vi "API - Get Rx Channels.vi"(7 "MCLB":refnum<vi>, 8 "error in (no error)":errorcluster, 11 "Node Ptr":T1 format="%.0x") -> (0 "error out":errorcluster, 3 "Node Ptr out":T1 format="%.0x", 5 "Channel Info":string[][](array[string]))   [LabVIEW 2016, in "UDP-Custom-Device System Explorer.lvlib"]
uses:
  UDP-Custom-Device System Explorer.lvlib
  <vilib>/NI Veristand/Custom Device API/Custom Device Item Ref.ctl
  Types/Channel Data Type.ctl
  Shared/Constants.vi
  <vilib>/NI Veristand/Custom Device API/Get Item Property (U16).vi
  <vilib>/NI VeriStand/Custom Device API/Custom Device API.lvlib
  Shared/UDP-Custom-Device Shared.lvlib
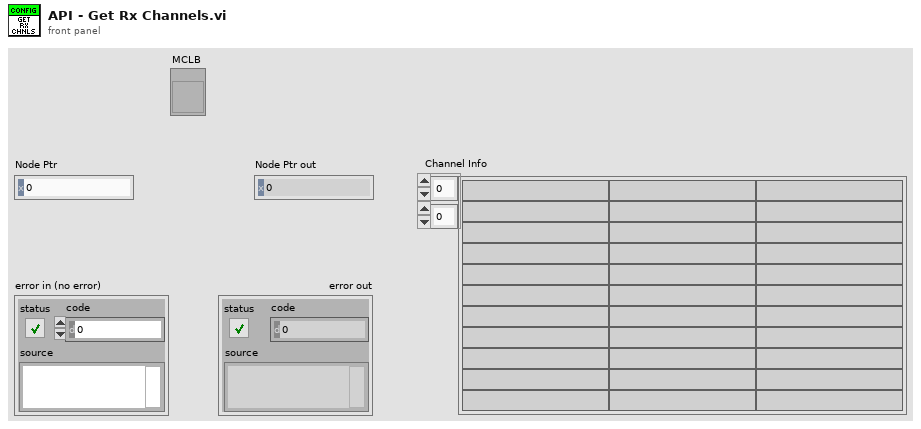
[diagram p1: front panel]
types:
  T1 = typedef "Custom Device API.lvlib/Custom Device Item Ref.ctl" = u64
  T2 = typedef "Custom Device API.lvlib/Custom Device Item Info.ctl" = cluster{"Name":string, "Is Channel":bool, "GUID":string, "Is Waveform":bool}
  T3 = typedef "UDP-Custom-Device System Explorer.lvlib/Channel Data Type.ctl" = enum16{"Boolean", "Single"}
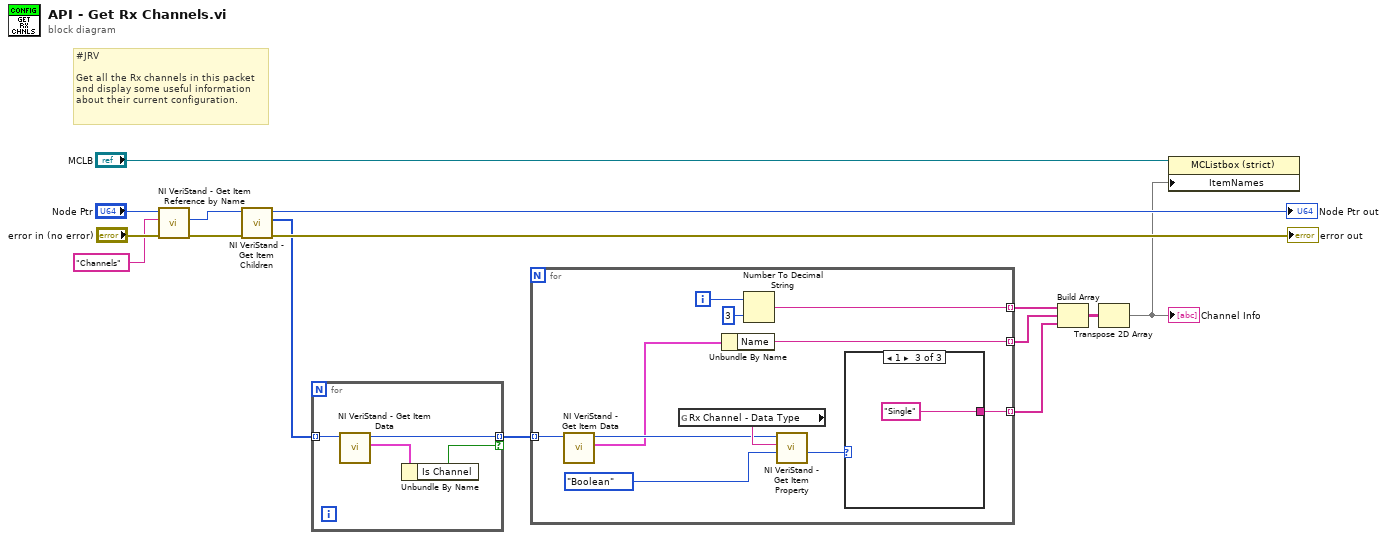
[diagram p0: block diagram]
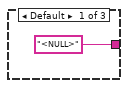
[diagram p2: hidden frame]
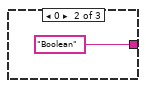
[diagram p3: hidden frame]
diagram:
  # "#JRV\n\nGet all the Rx channels in this packet\nand display some useful information\nabout their current configuration."
  n1 = call <vilib>:"NI VeriStand - Get Item Reference by Name.vi"("error in (no error)"="error in (no error)", "Item Name"="Channels" ("Section Name"), "Parent Ref in"="Node Ptr") -> ("error out"=w2:errorcluster, "Item Ref"=w4:T1)  [unwired: 5 in, 2 out]
  n2 = call <vilib>:"NI VeriStand - Get Item Children.vi"("error in (no error)"=w2, "Item Ref in"=w4) -> ("error out"=→"error out":errorcluster, "Child Refs"=w6:T1[], "Item Ref out"=→"Node Ptr out":T1)  [unwired: 6 in, 1 out]
  n3 = for {
    tunnel: [w18] -> w7 mode=indexing if=w16
    tunnel: w6 -> [w19] mode=indexing
    n4 = call <vilib>:"NI VeriStand - Get Item Data.vi"("Item Ref in"=w19) -> ("Item Info"=w17:T2, "Item Ref out"=w18:T1)  [unwired: 7 in, 2 out]
    n5 = Unbundle By Name(w17) -> ("Is Channel"=w16:bool)
  }
  n6 = for {
    tunnel: w7 -> [w29] mode=indexing
    tunnel: [w25] -> w11 mode=indexing
    tunnel: [w21] -> w12 mode=indexing
    tunnel: [w20] -> w13 mode=indexing
    i -> [w23]
    n7 = call <vilib>:"NI VeriStand - Get Item Data.vi"("Item Ref in"=w29) -> ("Item Info"=w24:T2, "Item Ref out"=w28:T1)  [unwired: 7 in, 2 out]
    n8 = global read "Constants.vi" "Rx Channel - Data Type"() -> (w30:string)
    n9 = Unbundle By Name(w24) -> ("Name"=w21:string)
    n10 = Number To Decimal String(number=w23, width (-)=i16 3) -> (decimal integer string=w20:string)
    n11 = call-poly <vilib>:"NI VeriStand - Get Item Property.vi"("Default Value"=Channel_Data_Type."Boolean" ("Data Type"), "Property Name"=w30, "Item Ref in"=w28) -> ("Value"=w26:u16)  [unwired: 5 in, 3 out]
    n12 = case shown="1" w26 {
      tunnel: ["<NULL>" "Boolean" "Single"] -> w25
      frame Default {
      }
      frame 0 {
      }
      frame 1 {
      }
    }
  }
  n13 = Build Array(w13, w12, w11) -> (w9:string[][])
  n14 = Transpose 2D Array(2D array=w9) -> (transposed array=w8:string[][])
  "Channel Info" <- w8
  n15 = property class="MCListbox (strict)"(reference="MCLB", "ItemNames"=w8) -> ()  [unwired: 1 in, 2 out]
